vi "Export_to_Excel.vi"(4 "Error In":errorcluster, 5 "Incoming data":string[][](array[string]), 7 "Export path":path=path "C:/temp/result.csv") -> (0 "Error Out":errorcluster, 3 "New path":path)   [LabVIEW 2018]
uses:
  <vilib>/Utility/file.llb/Write Delimited Spreadsheet (string).vi
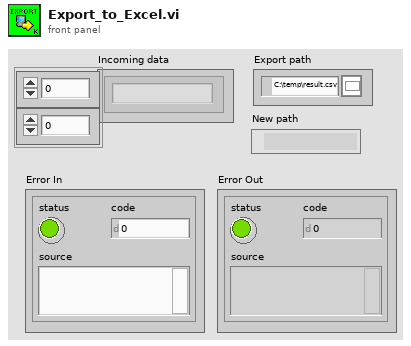
[diagram p1: front panel]
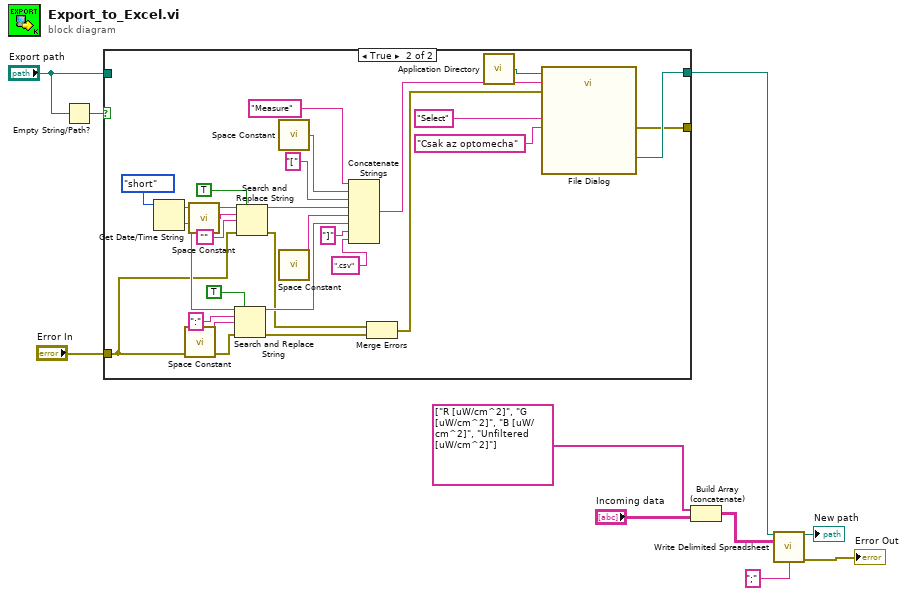
[diagram p0: block diagram]
diagram:
  n1 = Empty String/Path?(string/path="Export path") -> (empty?=w5:bool)
  n2 = case shown="True" w5 {
    tunnel: "Export path" -> [w12 _]
    tunnel: [w12 w19] -> w2
    tunnel: "Error In" -> [w11 w15]
    tunnel: [w11 w14] -> _
    frame False {
    }
    frame True {
      n3 = Get Date/Time String(date format (0)=enum16{"short", "long", "abbreviated"}."short") -> (date string=w35:string, time string=w32:string)  [unwired: 2 in]
      n4 = call <vilib>:"Space Constant.vi"() -> ("String"=w33:string)
      n5 = call <vilib>:"Space Constant.vi"() -> ("String"=w36:string)
      n6 = Search and Replace String(replace all?=TRUE ("replace all? (F)"), input string=w32, search string=":", replace string=w33, error in=w15) -> (result string=w34:string, error out=w16:errorcluster)  [unwired: 3 in, 2 out]
      n7 = Search and Replace String(replace all?=TRUE ("replace all? (F)"), input string=w35, search string=w36, replace string="", error in=w15) -> (result string=w37:string, error out=w17:errorcluster)  [unwired: 3 in, 2 out]
      n8 = call <vilib>:"Space Constant.vi"() -> ("String"=w38:string)
      n9 = call <vilib>:"Space Constant.vi"() -> ("String"=w31:string)
      n10 = Concatenate Strings("Measure", w38, "[", w37, w31, w34, "]", ".csv") -> (w22:string)
      n11 = Merge Errors(w17, w16) -> (w18:errorcluster)
      n12 = call <vilib>:"Application Directory.vi"() -> ("Application Directory"=w39:path)
      n13 = call "File Dialog"("start path"=w39, "prompt"="Csak az optomecha", "button label"="Select", "default name"=w22, "error in"=w18) -> ("selected path"=w19:path, "error out"=w14:errorcluster)  [unwired: 7 in, 2 out]
    }
  }
  n14 = Build Array (concatenate)(string[] ["R [uW/cm^2]", "G [uW/cm^2]", "B [uW/cm^2]", "Unfiltered [uW/cm^2]"] ("column headers"), "Incoming data") -> (w6:string[][])
  n15 = call-poly <vilib>:"Write Delimited Spreadsheet.vi"("file path (dialog if empty)"=w2, "2D data"=w6, "delimiter (\\t)"=";" ("delimiter (\\t)")) -> ("new file path (Not A Path if cancelled)"=→"New path":path, "error out"=→"Error Out":errorcluster)  [unwired: 11 in]
